vi "ChildModule.Lock Controls.vi"(8 "error in (no error)":errorcluster, 10 "Lock Ctrls":bool, 11 "Module Name":string) -> (0 "error out":errorcluster)   [LabVIEW 2016]
uses:
  <vilib>/KATE/Queues/Queue Utils.lvlib
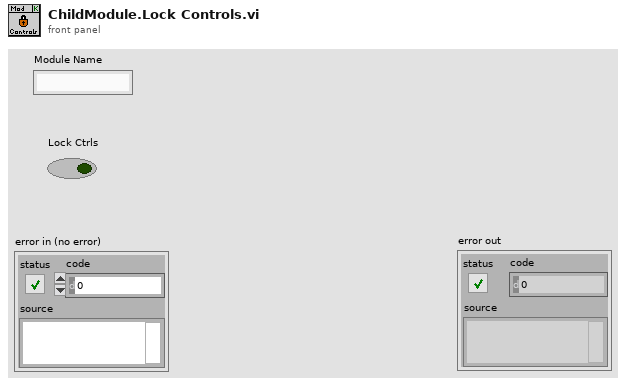
[diagram p1: front panel]
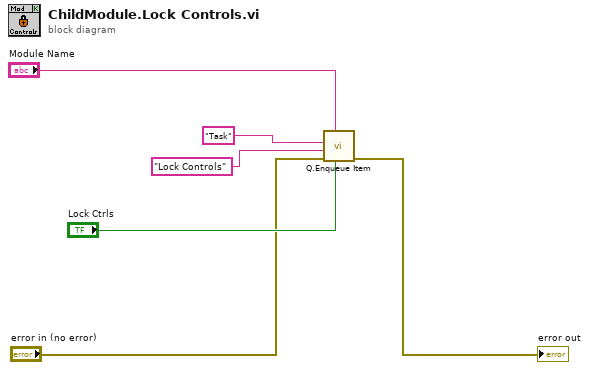
[diagram p0: block diagram]
diagram:
  n1 = call <vilib>:"Q.Enqueue Item.vi"("Data1"="Lock Ctrls", "Q Name"="Module Name", "Error In"="error in (no error)", "Sub"="Lock Controls" ("Cmd"), "Cmd"="Task") -> ("error out"=→"error out":errorcluster)  [unwired: 5 in, 1 out]
